vi "HFRR ADV v018 new software.vi"() -> ()   [LabVIEW 2025] (continued)
                }
                frame 126, Default {
                }
              }
            }
          }
          frame #1 {
            w4472 = TRUE ("Visible")
            n3478 = local read "S 91"() -> (w4489:string)
            n3479 = local read "S 90"() -> (w4488:string)
            n3480 = local read "S 88"() -> (w4487:string)
            n3481 = property on="File Path" class="Path"("Caption.Text"=w4488) -> ()  [unwired: 2 in, 2 out]
            n3482 = property on="SrvM CP" class="Bool (strict)"("Boolean Text.Text"=w4487) -> ()  [unwired: 2 in, 2 out]
            n3483 = local read "S 71"() -> (w4482:string)
            n3484 = local read "S 86"() -> (w4484:string)
            n3485 = local read "S 85"() -> (w4485:string)
            n3486 = local read "S 87"() -> (w4483:string)
            n3487 = local read "S 84"() -> (w4486:string)
            n3488 = local read "S 103"() -> (w4471:string)
            n3489 = local read "S 104"() -> (w4470:string)
            n3490 = property on="ENTER THE NEW PASSWORD" class="Str"("Caption.Text"=w4483) -> ()  [unwired: 2 in, 2 out]
            n3491 = property on="Password" class="Str"("Caption.Text"=w4485) -> ()  [unwired: 2 in, 2 out]
            n3492 = property on="ENTER CURRENT PASSWORD" class="Str"("Caption.Text"=w4484) -> ()  [unwired: 2 in, 2 out]
            n3493 = property on="EDIT" class="Bool (strict)"("Boolean Text.Text"=w4482) -> ()  [unwired: 2 in, 2 out]
            n3494 = property on="SAVE" class="Bool (strict)"("Boolean Text.Text"=w4486) -> ()  [unwired: 2 in, 2 out]
            n3495 = Build Array(w4471, w4470) -> (w4469:string[])
            n3496 = property on="Heater Button" class="Bool (strict)"("Strings [4]"=w4469) -> ()  [unwired: 2 in, 2 out]
            n3497 = property on="CH-HUMIDITY WET" class="DigNum (strict)"("Caption.Size to Text?"=w4472) -> ()  [unwired: 2 in, 2 out]
            n3498 = property on="CH-HUMIDITY DRY" class="DigNum (strict)"("Caption.Size to Text?"=w4472) -> ()  [unwired: 2 in, 2 out]
            n3499 = property on="CH-POWER -" class="DigNum (strict)"("Caption.Size to Text?"=w4472) -> ()  [unwired: 2 in, 2 out]
            n3500 = property on="CH-HEATER" class="DigNum (strict)"("Caption.Size to Text?"=w4472) -> ()  [unwired: 2 in, 2 out]
            n3501 = property on="CH-POWER +" class="DigNum (strict)"("Caption.Size to Text?"=w4472) -> ()  [unwired: 2 in, 2 out]
            n3502 = local read "S 92"() -> (w4481:string)
            n3503 = local read "S 93"() -> (w4480:string)
            n3504 = local read "S 105"() -> (w4467:string)
            n3505 = local read "S 106"() -> (w4466:string)
            n3506 = Build Array(w4481, w4480) -> ()  [unwired: 1 out]
            n3507 = Build Array(w4467, w4466) -> (w4468:string[])
            n3508 = local read "S 95"() -> (w4478:string)
            n3509 = local read "S 94"() -> (w4479:string)
            n3510 = local read "bs"() -> (w4494:string)
            n3511 = local read "as"() -> (w4495:string)
            n3512 = property on="Humidity" class="Bool (strict)"("Strings [4]"=w4468) -> ()  [unwired: 2 in, 2 out]
            n3513 = Concatenate Strings(w4494, "\r", w4495) -> ()  [unwired: 1 out]
            n3514 = property on="STROKE GAIN :" class="DigNum (strict)"("Caption.Text"=w4478) -> ()  [unwired: 2 in, 2 out]
            n3515 = property on="DISPLACEMENT :" class="DigNum (strict)"("Caption.Text"=w4479) -> ()  [unwired: 2 in, 2 out]
            n3516 = property on="Rh After" class="DigNum (strict)"("Caption.Size to Text?"=TRUE ("Caption.Size to Text")) -> ()  [unwired: 2 in, 2 out]
            n3517 = local read "S 48"() -> (w4518:string)
            n3518 = local read "S 50"() -> (w4516:string)
            n3519 = local read "S 51"() -> (w4515:string)
            n3520 = local read "S 49"() -> (w4517:string)
            n3521 = local read "S 52"() -> (w4514:string)
            n3522 = local read "as"() -> (w4499:string)
            n3523 = local read "bs"() -> (w4500:string)
            n3524 = local read "S 56"() -> (w4513:string)
            n3525 = local read "S 57"() -> (w4512:string)
            n3526 = local read "S 58"() -> (w4511:string)
            n3527 = local read "S 59"() -> (w4510:string)
            n3528 = property on="OPEN" class="Bool (strict)"("Boolean Text.Text"=w4514) -> ()  [unwired: 2 in, 2 out]
            n3529 = property on="OPEN 1" class="Bool (strict)"("Boolean Text.Text"=w4518) -> ()  [unwired: 2 in, 2 out]
            n3530 = property on="OPEN 2" class="Bool (strict)"("Boolean Text.Text"=w4517) -> ()  [unwired: 2 in, 2 out]
            n3531 = property on="OPEN 3" class="Bool (strict)"("Boolean Text.Text"=w4516) -> ()  [unwired: 2 in, 2 out]
            n3532 = property on="OPEN 4" class="Bool (strict)"("Boolean Text.Text"=w4515) -> ()  [unwired: 2 in, 2 out]
            n3533 = Concatenate Strings(w4500, "\r", w4499) -> ()  [unwired: 1 out]
            n3534 = local read "S 102"() -> (w4473:string)
            n3535 = property on="КОФ1" class="DigNum (strict)"("Caption.Text"=w4513) -> ()  [unwired: 2 in, 2 out]
            n3536 = local read "S 98"() -> (w4477:string)
            n3537 = local read "S 99"() -> (w4476:string)
            n3538 = local read "S 100"() -> (w4475:string)
            n3539 = local read "S 101"() -> (w4474:string)
            n3540 = property on="КОФ2" class="DigNum (strict)"("Caption.Text"=w4512) -> ()  [unwired: 2 in, 2 out]
            n3541 = property on="КОФ3" class="DigNum (strict)"("Caption.Text"=w4511) -> ()  [unwired: 2 in, 2 out]
            n3542 = property on="КОФ4" class="DigNum (strict)"("Caption.Text"=w4510) -> ()  [unwired: 2 in, 2 out]
            n3543 = local read "bs"() -> (w4498:string)
            n3544 = local read "as"() -> (w4497:string)
            n3545 = property on="CH-POWER +" class="DigNum (strict)"("Caption.Text"=w4477) -> ()  [unwired: 2 in, 2 out]
            n3546 = property on="CH-POWER -" class="DigNum (strict)"("Caption.Text"=w4476) -> ()  [unwired: 2 in, 2 out]
            n3547 = property on="CH-HEATER" class="DigNum (strict)"("Caption.Text"=w4475) -> ()  [unwired: 2 in, 2 out]
            n3548 = property on="CH-HUMIDITY DRY" class="DigNum (strict)"("Caption.Text"=w4474) -> ()  [unwired: 2 in, 2 out]
            n3549 = property on="CH-HUMIDITY WET" class="DigNum (strict)"("Caption.Text"=w4473) -> ()  [unwired: 2 in, 2 out]
            n3550 = local read "S 60"() -> (w4509:string)
            n3551 = local read "S 54"() -> (w4519:string)
            n3552 = Concatenate Strings(w4498, "\r", w4497) -> ()  [unwired: 1 out]
            n3553 = Concatenate Strings(w4519, w4509) -> ()  [unwired: 1 out]
            n3554 = local read "S 77"() -> (→"String 43":string)
            n3555 = local read "S 76"() -> (w4492:string)
            n3556 = local read "S 78"() -> (w4491:string)
            n3557 = local read "S 71"() -> (w4503:string)
            n3558 = local read "S 66"() -> (w4508:string)
            n3559 = local read "S 67"() -> (w4507:string)
            n3560 = local read "S 68"() -> (w4506:string)
            n3561 = local read "S 69"() -> (w4505:string)
            n3562 = local read "S 70"() -> (w4504:string)
            n3563 = property on="AIR TEMP" class="DigNum (strict)"("Caption.Text"=w4491) -> ()  [unwired: 2 in, 2 out]
            n3564 = property on="Set Strk" class="DigNum (strict)"("Caption.Text"=w4492) -> ()  [unwired: 2 in, 2 out]
            n3565 = property on="FRIC. FORCE :" class="DigNum (strict)"("Caption.Text"=w4508) -> ()  [unwired: 2 in, 2 out]
            n3566 = property on="TEMPERATURE :" class="DigNum (strict)"("Caption.Text"=w4507) -> ()  [unwired: 2 in, 2 out]
            n3567 = property on="SPEED OUT:" class="DigNum (strict)"("Caption.Text"=w4506) -> ()  [unwired: 2 in, 2 out]
            n3568 = property on="AIR TEMPERATURE :" class="DigNum (strict)"("Caption.Text"=w4505) -> ()  [unwired: 2 in, 2 out]
            n3569 = property on="HUMIDITY:" class="DigNum (strict)"("Caption.Text"=w4504) -> ()  [unwired: 2 in, 2 out]
            n3570 = property on="EDIT" class="Bool (strict)"("Boolean Text.Text"=w4503) -> ()  [unwired: 2 in, 2 out]
            n3571 = local read "S 79"() -> (w4490:string)
          }
          frame #2 {
          }
        }
        n3572 = local write "Lan flag"(10.0 ("Lan flag")) -> ()
      }
      frame Enabled {
      }
    }
    n3573 = Wait (ms)(milliseconds to wait=u32 2000) -> ()  [unwired: 1 out]
    n3574 = local read "Quit"() -> (w4293:bool)
  }
  n3575 = while {
    shift-right: [w4525] -> _
    shift-left: _ -> [w4526]
    shift-right: [w4523] -> _
    shift-left: T18 {"Read Heave and Surge"="", "Bytes at Heave Port"=0.0, "Heave and Surge COM Port:"="COM9", "Com Port 2"="COM7", "Residual Due"="", "Heave COM Status 2"=TRUE, "Heave COM Status"=TRUE, "Port 2"=TRUE, "Sway PPR"=6400.0, "Surge PPR"=6400.0, "Heave PPR"=6400.0, "Sway Pitch"=2.0, "Surge Pitch"=3.0, "Heave Pitch"=4.0, "Sway Pulses/mm"=320.0, "Surge Pulses/mm"=1600.0, "Heave Pulses/mm"=1600.0, "inner loop"=0.0, "Read Heave and Surge 2"="", "String 36"="", "Write S"=FALSE, "WriteCC1"=[""], "Heave COM Loop"=0, "LastCom"="", "EXIT"=FALSE, "Error Heave"={"status"=TRUE, "code"=-1073807343, "source"=""}} -> [w4522]
    shift-right: [w4520] -> _
    shift-left: enum16{"init", "MAIN", "Panel Close"}."init" -> [w4521]
    stop <- w4524 stop-if-true
    n3576 = case shown="\"init\"" w4521 {
      tunnel: w4526 -> [w4540 w4556 w4616 w4618]
      tunnel: [w4535 w4564 w4616 w4618] -> w4525
      tunnel: [_ _ TRUE _] -> w4524
      tunnel: [w4531 w4562 w4614 w4617] -> w4523
      tunnel: w4522 -> [w4537 w4555 w4614 w4617]
      tunnel: [enum16{"init", "MAIN", "Panel Close"}."MAIN" w4550 _ _] -> w4520
      frame "init" {
        n3577 = local read "Com Port 1"() -> (w4527:refnum<visa-resource-name>)
        n3578 = Bundle By Name(cluster=w4537, "Heave and Surge COM Port:"=w4527) -> (w4536:T18)
        n3579 = call "Instrument fgv uno.vi"("Enum"=T31."INIT", "error in (no error) 2"=w4540, "INPUT"=w4536) -> ("error"=w4538:errorcluster, "output"=w4534:T18)  [unwired: 6 in, 1 out]
        n3580 = case shown="Error" w4538 {
          selector: w4538 -> [w4542 _]
          tunnel: [w4542 w4546] -> w4535
          tunnel: w4534 -> [w4541 w4544]
          tunnel: [w4541 w4543] -> w4532
          frame No Error {
          }
          frame Error {
            n3581 = call "Instrument fgv uno.vi"("Enum"=T31."ERROR INIT", "INPUT"=w4544) -> ("error"=w4547:errorcluster, "output"=w4543:T18)  [unwired: 7 in, 1 out]
            n3582 = call <vilib>:"Clear Errors.vi"("error in (no error)"=w4547) -> ("error out"=w4546:errorcluster)  [unwired: 5 in, 1 out]
          }
        }
        n3583 = local read "LastCom 2"() -> (w4530:string)
        n3584 = Unbundle By Name(w4532) -> ("Heave COM Status 2"=→"COM Status 2" →"Instrument Status 2":bool, "Error Heave"=→"Error  2":errorcluster)  [unwired: 1 out]
        n3585 = Bundle By Name(cluster=w4532, "LastCom"=w4530) -> (w4531:T18)
      }
      frame "MAIN" {
        n3586 = Unbundle By Name(w4555) -> ("Com Port 2"=w4566:refnum<visa-resource-name>)
        n3587 = local read "Com Port 1"() -> (w4549:refnum<visa-resource-name>)
        n3588 = local write "Com Port 5"(w4566) -> ()
        n3589 = Bundle By Name(cluster=w4555, "Heave and Surge COM Port:"=w4549) -> (w4554:T18)
        n3590 = Equal?(x=w4566, y=w4549) -> (x = y?=w4565:bool)
        n3591 = case shown="True" w4565 {
          tunnel: [w4570 w4587] -> w4564
          tunnel: w4556 -> [w4571 w4593]
          tunnel: w4554 -> [w4569 w4591]
          tunnel: [w4568 w4586] -> w4562
          frame False {
            n3592 = call <vilib>:"Clear Errors.vi"("error in (no error)"=w4571) -> ("error out"=w4567:errorcluster)  [unwired: 5 in, 1 out]
            n3593 = call "Instrument fgv uno.vi"("Enum"=T31."ERROR INIT", "error in (no error) 2"=w4567, "INPUT"=w4569) -> ("error"=w4573:errorcluster, "output"=w4568:T18)  [unwired: 6 in, 1 out]
            n3594 = call <vilib>:"Clear Errors.vi"("error in (no error)"=w4573) -> ("error out"=w4570:errorcluster)  [unwired: 5 in, 1 out]
          }
          frame True {
            n3595 = call "Instrument fgv uno.vi"("Enum"=T31."READ", "error in (no error) 2"=w4593, "INPUT"=w4591) -> ("error"=w4592:errorcluster, "output"=w4583:T18)  [unwired: 6 in, 1 out]
            n3596 = Bundle By Name(cluster=w4583, "String 36"="String 15") -> (w4582:T18)
            n3597 = case shown="True" "Write S 2" {
              selector: "Write S 2" -> [_ w4613]
              tunnel: w4592 -> [w4606 w4612]
              tunnel: [w4606 w4611] -> w4579
              tunnel: w4582 -> [w4605 w4608]
              tunnel: [w4605 w4607] -> w4578
              frame False {
              }
              frame True {
                n3598 = Not(x=w4613) -> (.not. x?=w4609:bool)
                n3599 = local write "Write S 2"(w4609) -> ()
                n3600 = call "Instrument fgv uno.vi"("Enum"=T31."MANUAL WRITE", "error in (no error) 2"=w4612, "INPUT"=w4608) -> ("error"=w4611:errorcluster, "output"=w4607:T18)  [unwired: 6 in, 1 out]
              }
            }
            n3601 = Array Size(array="WriteHumidity 2") -> (size(s)=w4576:i32)
            n3602 = Greater Than 0?(x=w4576) -> (x > 0?=w4574:bool)
            n3603 = call "Instrument fgv uno.vi"("Enum"=T31."WRITE", "error in (no error) 2"=w4579, "WriteCC1"="WriteHumidity 2", "INPUT"=w4578) -> ("error"=w4589:errorcluster, "WriteCC1 2"=w4577:string[], "output"=w4588:T18)  [unwired: 5 in]
            n3604 = case shown="True" w4574 {
              tunnel: w4577 -> [_ w4595]
              frame False {
              }
              frame True {
                n3605 = local write "WriteHumidity 2"(w4595) -> ()
              }
            }
            n3606 = case shown="No Error" w4589 {
              selector: w4589 -> [w4596 w4599]
              tunnel: w4588 -> [w4597 w4604]
              tunnel: [w4597 w4603] -> w4586
              tunnel: [w4596 w4601] -> w4587
              frame No Error {
              }
              frame Error {
                n3607 = call <vilib>:"Clear Errors.vi"("error in (no error)"=w4599) -> ("error out"=w4598:errorcluster)  [unwired: 5 in, 1 out]
                n3608 = call "Instrument fgv uno.vi"("Enum"=T31."ERROR INIT", "error in (no error) 2"=w4598, "INPUT"=w4604) -> ("error"=w4602:errorcluster, "output"=w4603:T18)  [unwired: 6 in, 1 out]
                n3609 = call <vilib>:"Clear Errors.vi"("error in (no error)"=w4602) -> ("error out"=w4601:errorcluster)  [unwired: 5 in, 1 out]
              }
            }
            n3610 = Unbundle By Name(w4586) -> ("LastCom"=→"LastCom 2":string, "Read Heave and Surge"=→"Read Uno":string)
          }
        }
        n3611 = Unbundle By Name(w4562) -> ("Heave COM Status 2"=w4563:bool, "Heave COM Status"=w4548:bool, "Error Heave"=w4560:errorcluster, "Bytes at Heave Port"=→"Bytes at Humidity Port  2":dbl)
        n3612 = Unbundle By Name(w4560) -> ("status"=→"Humidity Port 2":bool)
        n3613 = Not(x=w4548) -> (.not. x?=w4557:bool)
        n3614 = local write "Error  2"(w4560) -> ()
        n3615 = Not(x=w4563) -> (.not. x?=w4558:bool)
        n3616 = local write "Instrument Status 2"(w4557) -> ()
        n3617 = local write "COM Status 2"(w4558) -> ()
        n3618 = local write "Port 1a"(w4548) -> ()
        n3619 = local read "Quit"() -> (w4551:bool)
        n3620 = Select(t=enum16{"init", "MAIN", "Panel Close"}."Panel Close", s=w4551, f=enum16{"init", "MAIN", "Panel Close"}."MAIN") -> (s? t:f=w4550:enum16{"init", "MAIN", "Panel Close"})
      }
      frame "Panel Close" {
      }
      frame Default {
      }
    }
  }
  n3621 = disable-structure shown="Disabled" {
    frame Disabled {
      n3622 = while {
        tunnel: [w4620] -> _
        i -> [w4620]
        stop <- w4619 continue-if-true
        n3623 = Wait (ms)(milliseconds to wait=u32 50) -> ()  [unwired: 1 out]
        n3624 = stacked-sequence {
          frame #0 {
            # "Controls Text color"
            # "Controls BG color"
            n3625 = property on="FILE" class="Str"("Text.Text Colors:Text Color"="SC  Text") -> ()  [unwired: 2 in, 2 out]
            n3626 = property on="Fuel Discription :" class="Str"("Text.Text Colors:Text Color"="SC  Text") -> ()  [unwired: 2 in, 2 out]
            n3627 = property on="tested by" class="Str"("Text.Text Colors:Text Color"="SC  Text") -> ()  [unwired: 2 in, 2 out]
            n3628 = property on="Remarks :" class="Str"("Text.Text Colors:Text Color"="SC  Text") -> ()  [unwired: 2 in, 2 out]
            n3629 = property class="DigNum (strict)"("Numeric Text.Text Colors:BG Color"="NC BG") -> ()  [unwired: 2 in, 2 out]
            n3630 = property class="DigNum (strict)"("Numeric Text.Text Colors:BG Color"="NC BG") -> ()  [unwired: 2 in, 2 out]
            n3631 = property class="DigNum (strict)"("Numeric Text.Text Colors:BG Color"="NC BG") -> ()  [unwired: 2 in, 2 out]
            n3632 = property class="DigNum (strict)"("Numeric Text.Text Colors:BG Color"="NC BG") -> ()  [unwired: 2 in, 2 out]
            n3633 = property class="DigNum (strict)"("Numeric Text.Text Colors:BG Color"="NC BG") -> ()  [unwired: 2 in, 2 out]
            n3634 = property class="DigNum (strict)"("Numeric Text.Text Colors:BG Color"="NC BG") -> ()  [unwired: 2 in, 2 out]
            n3635 = property class="DigNum (strict)"("Numeric Text.Text Colors:BG Color"="NC BG") -> ()  [unwired: 2 in, 2 out]
            n3636 = property class="DigNum (strict)"("Numeric Text.Text Colors:BG Color"="NC BG") -> ()  [unwired: 2 in, 2 out]
            n3637 = property class="DigNum (strict)"("Numeric Text.Text Colors:BG Color"="NC BG") -> ()  [unwired: 2 in, 2 out]
            n3638 = property class="DigNum (strict)"("Numeric Text.Text Colors:BG Color"="NC BG") -> ()  [unwired: 2 in, 2 out]
            n3639 = property class="DigNum (strict)"("Numeric Text.Text Colors:BG Color"="NC BG") -> ()  [unwired: 2 in, 2 out]
            n3640 = property class="DigNum (strict)"("Numeric Text.Text Colors:BG Color"="NC BG") -> ()  [unwired: 2 in, 2 out]
            n3641 = property on="FILE" class="Str"("Text.Text Colors:BG Color"="SC BG 3") -> ()  [unwired: 2 in, 2 out]
            n3642 = property on="Fuel Discription :" class="Str"("Text.Text Colors:BG Color"="SC BG 3") -> ()  [unwired: 2 in, 2 out]
            n3643 = property on="tested by" class="Str"("Text.Text Colors:BG Color"="SC BG 3") -> ()  [unwired: 2 in, 2 out]
            n3644 = property on="Remarks :" class="Str"("Text.Text Colors:BG Color"="SC BG 3") -> ()  [unwired: 2 in, 2 out]
            n3645 = property class="DigNum (strict)"("Numeric Text.Text Colors:Text Color"="NC Text") -> ()  [unwired: 2 in, 2 out]
            n3646 = property class="DigNum (strict)"("Numeric Text.Text Colors:Text Color"="NC Text") -> ()  [unwired: 2 in, 2 out]
            n3647 = property class="DigNum (strict)"("Numeric Text.Text Colors:Text Color"="NC Text") -> ()  [unwired: 2 in, 2 out]
            n3648 = property class="DigNum (strict)"("Numeric Text.Text Colors:Text Color"="NC Text") -> ()  [unwired: 2 in, 2 out]
            n3649 = property class="DigNum (strict)"("Numeric Text.Text Colors:Text Color"="NC Text") -> ()  [unwired: 2 in, 2 out]
            n3650 = property class="DigNum (strict)"("Numeric Text.Text Colors:Text Color"="NC Text") -> ()  [unwired: 2 in, 2 out]
            n3651 = property class="DigNum (strict)"("Numeric Text.Text Colors:Text Color"="NC Text") -> ()  [unwired: 2 in, 2 out]
            n3652 = property class="DigNum (strict)"("Numeric Text.Text Colors:Text Color"="NC Text") -> ()  [unwired: 2 in, 2 out]
            n3653 = property class="DigNum (strict)"("Numeric Text.Text Colors:Text Color"="NC Text") -> ()  [unwired: 2 in, 2 out]
            n3654 = property class="DigNum (strict)"("Numeric Text.Text Colors:Text Color"="NC Text") -> ()  [unwired: 2 in, 2 out]
            n3655 = property class="DigNum (strict)"("Numeric Text.Text Colors:Text Color"="NC Text") -> ()  [unwired: 2 in, 2 out]
            n3656 = property class="DigNum (strict)"("Numeric Text.Text Colors:Text Color"="NC Text") -> ()  [unwired: 2 in, 2 out]
            n3657 = property class="DigNum (strict)"("Numeric Text.Text Colors:Text Color"="NI Text  2") -> ()  [unwired: 2 in, 2 out]
            n3658 = property class="DigNum (strict)"("Numeric Text.Text Colors:Text Color"="NI Text  2") -> ()  [unwired: 2 in, 2 out]
            n3659 = property class="DigNum (strict)"("Numeric Text.Text Colors:Text Color"="NI Text  2") -> ()  [unwired: 2 in, 2 out]
            n3660 = property class="DigNum (strict)"("Numeric Text.Text Colors:Text Color"="NI Text  2") -> ()  [unwired: 2 in, 2 out]
            n3661 = property class="DigNum (strict)"("Numeric Text.Text Colors:Text Color"="NI Text  2") -> ()  [unwired: 2 in, 2 out]
            n3662 = property class="DigNum (strict)"("Numeric Text.Text Colors:Text Color"="NI Text  2") -> ()  [unwired: 2 in, 2 out]
            n3663 = property class="DigNum (strict)"("Numeric Text.Text Colors:Text Color"="NI Text  2") -> ()  [unwired: 2 in, 2 out]
            n3664 = property class="DigNum (strict)"("Numeric Text.Text Colors:Text Color"="NI Text  2") -> ()  [unwired: 2 in, 2 out]
            n3665 = property class="DigNum (strict)"("Numeric Text.Text Colors:Text Color"="NI Text  2") -> ()  [unwired: 2 in, 2 out]
            n3666 = property class="DigNum (strict)"("Numeric Text.Text Colors:Text Color"="NI Text  2") -> ()  [unwired: 2 in, 2 out]
            n3667 = property class="DigNum (strict)"("Numeric Text.Text Colors:Text Color"="NI Text  2") -> ()  [unwired: 2 in, 2 out]
            n3668 = property class="DigNum (strict)"("Numeric Text.Text Colors:Text Color"="NI Text  2") -> ()  [unwired: 2 in, 2 out]
            n3669 = property class="DigNum (strict)"("Numeric Text.Text Colors:Text Color"="NI Text  2") -> ()  [unwired: 2 in, 2 out]
            n3670 = property class="DigNum (strict)"("Numeric Text.Text Colors:Text Color"="NI Text  2") -> ()  [unwired: 2 in, 2 out]
            n3671 = property class="DigNum (strict)"("Numeric Text.Text Colors:Text Color"="NI Text  2") -> ()  [unwired: 2 in, 2 out]
            n3672 = property on="Coefficient Of Friction" class="XYGraph (strict)"("Plot Area:Colors:FG Color"="GFG  2", "Plot Area:Colors:BG Color"="GBG   2") -> ()  [unwired: 2 in, 2 out]
            n3673 = property on="Humidity ( %RH )" class="XYGraph (strict)"("Plot Area:Colors:FG Color"="GFG  2", "Plot Area:Colors:BG Color"="GBG   2") -> ()  [unwired: 2 in, 2 out]
            n3674 = property on="Air Temperature  ( °C )" class="XYGraph (strict)"("Plot Area:Colors:FG Color"="GFG  2", "Plot Area:Colors:BG Color"="GBG   2") -> ()  [unwired: 2 in, 2 out]
            n3675 = property on="Sample Temperature ( °C )" class="XYGraph (strict)"("Plot Area:Colors:FG Color"="GFG  2", "Plot Area:Colors:BG Color"="GBG   2") -> ()  [unwired: 2 in, 2 out]
            n3676 = property class="DigNum (strict)"("Numeric Text.Text Colors:BG Color"="NI BG 2") -> ()  [unwired: 2 in, 2 out]
            n3677 = property class="DigNum (strict)"("Numeric Text.Text Colors:BG Color"="NI BG 2") -> ()  [unwired: 2 in, 2 out]
            n3678 = property class="DigNum (strict)"("Numeric Text.Text Colors:BG Color"="NI BG 2") -> ()  [unwired: 2 in, 2 out]
            n3679 = property class="DigNum (strict)"("Numeric Text.Text Colors:BG Color"="NI BG 2") -> ()  [unwired: 2 in, 2 out]
            n3680 = property class="DigNum (strict)"("Numeric Text.Text Colors:BG Color"="NI BG 2") -> ()  [unwired: 2 in, 2 out]
            n3681 = property class="DigNum (strict)"("Numeric Text.Text Colors:BG Color"="NI BG 2") -> ()  [unwired: 2 in, 2 out]
            n3682 = property class="DigNum (strict)"("Numeric Text.Text Colors:BG Color"="NI BG 2") -> ()  [unwired: 2 in, 2 out]
            n3683 = property class="DigNum (strict)"("Numeric Text.Text Colors:BG Color"="NI BG 2") -> ()  [unwired: 2 in, 2 out]
            n3684 = property class="DigNum (strict)"("Numeric Text.Text Colors:BG Color"="NI BG 2") -> ()  [unwired: 2 in, 2 out]
            n3685 = property class="DigNum (strict)"("Numeric Text.Text Colors:BG Color"="NI BG 2") -> ()  [unwired: 2 in, 2 out]
            n3686 = property class="DigNum (strict)"("Numeric Text.Text Colors:BG Color"="NI BG 2") -> ()  [unwired: 2 in, 2 out]
            n3687 = property class="DigNum (strict)"("Numeric Text.Text Colors:BG Color"="NI BG 2") -> ()  [unwired: 2 in, 2 out]
            n3688 = property class="DigNum (strict)"("Numeric Text.Text Colors:BG Color"="NI BG 2") -> ()  [unwired: 2 in, 2 out]
            n3689 = property class="DigNum (strict)"("Numeric Text.Text Colors:BG Color"="NI BG 2") -> ()  [unwired: 2 in, 2 out]
            n3690 = property class="DigNum (strict)"("Numeric Text.Text Colors:BG Color"="NI BG 2") -> ()  [unwired: 2 in, 2 out]
            n3691 = property class="Bool"("Colors [4]"="Boolean BC T & BG") -> ()  [unwired: 2 in, 2 out]
            n3692 = property on="Save & Continue" class="Bool (strict)"("Colors [4]"="Boolean BC T & BG") -> ()  [unwired: 2 in, 2 out]
            n3693 = property on="Heater Button" class="Bool (strict)"("Colors [4]"="Boolean BC T & BG") -> ()  [unwired: 2 in, 2 out]
            n3694 = property class="Bool"("Colors [4]"="Boolean BC T & BG") -> ()  [unwired: 2 in, 2 out]
            n3695 = property on="Humidity" class="Bool (strict)"("Colors [4]"="Boolean BC T & BG") -> ()  [unwired: 2 in, 2 out]
            n3696 = property class="Bool (strict)"("Colors [4]"="Boolean BC T & BG") -> ()  [unwired: 2 in, 2 out]
            n3697 = property on="RUN" class="Bool (strict)"("Colors [4]"="Boolean BC T & BG") -> ()  [unwired: 2 in, 2 out]
            n3698 = property on="trip1 8" class="Bool (strict)"("Colors [4]"="Boolean BC T & BG") -> ()  [unwired: 2 in, 2 out]
            n3699 = property class="Bool"("Colors [4]"="Boolean BC T & BG") -> ()  [unwired: 2 in, 2 out]
            n3700 = property class="Bool (strict)"("Colors [4]"="Boolean BC T & BG") -> ()  [unwired: 2 in, 2 out]
            n3701 = property on="OPEN 1" class="Bool (strict)"("Colors [4]"="Boolean BC T & BG 2") -> ()  [unwired: 2 in, 2 out]
            n3702 = property on="OPEN 2" class="Bool (strict)"("Colors [4]"="Boolean BC T & BG 2") -> ()  [unwired: 2 in, 2 out]
            n3703 = property on="OPEN 3" class="Bool (strict)"("Colors [4]"="Boolean BC T & BG 2") -> ()  [unwired: 2 in, 2 out]
            n3704 = property on="OPEN 4" class="Bool (strict)"("Colors [4]"="Boolean BC T & BG 2") -> ()  [unwired: 2 in, 2 out]
            n3705 = property on="OPEN" class="Bool (strict)"("Colors [4]"="Boolean BC T & BG 2") -> ()  [unwired: 2 in, 2 out]
            n3706 = property on="rstv2" class="Bool"("Colors [4]"="Boolean BC T & BG 2") -> ()  [unwired: 2 in, 2 out]
            n3707 = property on="RST CP" class="Bool"("Colors [4]"="Boolean BC T & BG 2") -> ()  [unwired: 2 in, 2 out]
            n3708 = property on="RSTV1 3" class="Bool"("Colors [4]"="Boolean BC T & BG 2") -> ()  [unwired: 2 in, 2 out]
            n3709 = property on="RSTV1 2" class="Bool"("Colors [4]"="Boolean BC T & BG 2") -> ()  [unwired: 2 in, 2 out]
          }
          frame #1 {
          }
        }
        n3710 = local read "Quit"() -> (w4619:bool)
      }
    }
    frame Enabled {
    }
  }
  n3711 = while {
    shift-right: [w4637] -> _
    shift-left: _ -> [w4638]
    shift-right: [w4635] -> _
    shift-left: T18 {"Read Heave and Surge"="", "Bytes at Heave Port"=0.0, "Heave and Surge COM Port:"="COM9", "Com Port 2"="COM7", "Residual Due"="", "Heave COM Status 2"=TRUE, "Heave COM Status"=TRUE, "Port 2"=TRUE, "Sway PPR"=6400.0, "Surge PPR"=6400.0, "Heave PPR"=6400.0, "Sway Pitch"=2.0, "Surge Pitch"=3.0, "Heave Pitch"=4.0, "Sway Pulses/mm"=320.0, "Surge Pulses/mm"=1600.0, "Heave Pulses/mm"=1600.0, "inner loop"=0.0, "Read Heave and Surge 2"="", "String 36"="", "Write S"=FALSE, "WriteCC1"=[""], "Heave COM Loop"=0, "LastCom"="", "EXIT"=FALSE, "Error Heave"={"status"=TRUE, "code"=-1073807343, "source"=""}} -> [w4634]
    shift-right: [w4632] -> _
    shift-left: enum16{"init", "MAIN", "Panel Close"}."init" -> [w4633]
    stop <- w4636 stop-if-true
    n3712 = case shown="\"init\"" w4633 {
      tunnel: w4638 -> [w4652 w4667 w4728 w4730]
      tunnel: [w4646 w4676 w4728 w4730] -> w4637
      tunnel: [_ _ TRUE _] -> w4636
      tunnel: [w4642 w4673 w4726 w4729] -> w4635
      tunnel: w4634 -> [w4649 w4666 w4726 w4729]
      tunnel: [enum16{"init", "MAIN", "Panel Close"}."MAIN" w4660 _ _] -> w4632
      frame "init" {
        n3713 = Bundle By Name(cluster=w4649, "Heave and Surge COM Port:"="C3 :") -> (w4648:T18)
        n3714 = call "Instrument fgv.vi"("Enum"=T31."INIT", "error in (no error) 2"=w4652, "INPUT"=w4648) -> ("error"=w4650:errorcluster, "output"=w4645:T18)  [unwired: 6 in, 1 out]
        n3715 = case shown="Error" w4650 {
          selector: w4650 -> [w4654 _]
          tunnel: [w4654 w4658] -> w4646
          tunnel: w4645 -> [w4653 w4656]
          tunnel: [w4653 w4655] -> w4643
          frame No Error {
          }
          frame Error {
            n3716 = call "Instrument fgv.vi"("Enum"=T31."ERROR INIT", "INPUT"=w4656) -> ("error"=w4659:errorcluster, "output"=w4655:T18)  [unwired: 7 in, 1 out]
            n3717 = call <vilib>:"Clear Errors.vi"("error in (no error)"=w4659) -> ("error out"=w4658:errorcluster)  [unwired: 5 in, 1 out]
          }
        }
        n3718 = local read "LastCom"() -> (w4641:string)
        n3719 = Unbundle By Name(w4643) -> ("Heave COM Status 2"=→"COM Status" →"Instrument Status":bool, "Error Heave"=→"Error":errorcluster)  [unwired: 1 out]
        n3720 = Bundle By Name(cluster=w4643, "LastCom"=w4641) -> (w4642:T18)
      }
      frame "MAIN" {
        n3721 = Unbundle By Name(w4666) -> ("Com Port 2"=w4678:refnum<visa-resource-name>)
        n3722 = local write "Com Port 4"(w4678) -> ()
        n3723 = local read "C3 :"() -> (w4664:refnum<visa-resource-name>)
        n3724 = Bundle By Name(cluster=w4666, "Heave and Surge COM Port:"=w4664) -> (w4665:T18)
        n3725 = Equal?(x=w4678, y=w4664) -> (x = y?=w4677:bool)
        n3726 = case shown="True" w4677 {
          tunnel: [w4682 w4699] -> w4676
          tunnel: w4667 -> [w4683 w4705]
          tunnel: w4665 -> [w4681 w4703]
          tunnel: [w4680 w4698] -> w4673
          frame False {
            n3727 = call <vilib>:"Clear Errors.vi"("error in (no error)"=w4683) -> ("error out"=w4679:errorcluster)  [unwired: 5 in, 1 out]
            n3728 = call "Instrument fgv.vi"("Enum"=T31."ERROR INIT", "error in (no error) 2"=w4679, "INPUT"=w4681) -> ("error"=w4685:errorcluster, "output"=w4680:T18)  [unwired: 6 in, 1 out]
            n3729 = call <vilib>:"Clear Errors.vi"("error in (no error)"=w4685) -> ("error out"=w4682:errorcluster)  [unwired: 5 in, 1 out]
          }
          frame True {
            n3730 = call "Instrument fgv.vi"("Enum"=T31."READ", "error in (no error) 2"=w4705, "INPUT"=w4703) -> ("error"=w4704:errorcluster, "output"=w4695:T18)  [unwired: 6 in, 1 out]
            n3731 = Bundle By Name(cluster=w4695, "String 36"="String 11") -> (w4694:T18)
            n3732 = case shown="True" "Write S" {
              selector: "Write S" -> [_ w4725]
              tunnel: w4704 -> [w4718 w4724]
              tunnel: [w4718 w4723] -> w4691
              tunnel: w4694 -> [w4717 w4720]
              tunnel: [w4717 w4719] -> w4690
              frame False {
              }
              frame True {
                n3733 = Not(x=w4725) -> (.not. x?=w4721:bool)
                n3734 = local write "Write S"(w4721) -> ()
                n3735 = call "Instrument fgv.vi"("Enum"=T31."MANUAL WRITE", "error in (no error) 2"=w4724, "INPUT"=w4720) -> ("error"=w4723:errorcluster, "output"=w4719:T18)  [unwired: 6 in, 1 out]
              }
            }
            n3736 = Array Size(array="WriteHumidity") -> (size(s)=w4688:i32)
            n3737 = Greater Than 0?(x=w4688) -> (x > 0?=w4686:bool)
            n3738 = call "Instrument fgv.vi"("Enum"=T31."WRITE", "error in (no error) 2"=w4691, "WriteCC1"="WriteHumidity", "INPUT"=w4690) -> ("error"=w4701:errorcluster, "WriteCC1 2"=w4689:string[], "output"=w4700:T18)  [unwired: 5 in]
            n3739 = case shown="True" w4686 {
              tunnel: w4689 -> [_ w4707]
              frame False {
              }
              frame True {
                n3740 = local write "WriteHumidity"(w4707) -> ()
              }
            }
            n3741 = case shown="Error" w4701 {
              selector: w4701 -> [w4708 w4711]
              tunnel: w4700 -> [w4709 w4716]
              tunnel: [w4709 w4715] -> w4698
              tunnel: [w4708 w4713] -> w4699
              frame No Error {
              }
              frame Error {
                n3742 = call <vilib>:"Clear Errors.vi"("error in (no error)"=w4711) -> ("error out"=w4710:errorcluster)  [unwired: 5 in, 1 out]
                n3743 = call "Instrument fgv.vi"("Enum"=T31."ERROR INIT", "error in (no error) 2"=w4710, "INPUT"=w4716) -> ("error"=w4714:errorcluster, "output"=w4715:T18)  [unwired: 6 in, 1 out]
                n3744 = call <vilib>:"Clear Errors.vi"("error in (no error)"=w4714) -> ("error out"=w4713:errorcluster)  [unwired: 5 in, 1 out]
              }
            }
            n3745 = Unbundle By Name(w4698) -> ("LastCom"=→"LastCom":string, "Read Heave and Surge"=→"Read Humidity":string)
          }
        }
        n3746 = Unbundle By Name(w4673) -> ("Heave COM Status 2"=w4675:bool, "Heave COM Status"=w4674:bool, "Error Heave"=w4671:errorcluster, "Bytes at Heave Port"=→"Bytes at Humidity Port":dbl)
        n3747 = Unbundle By Name(w4671) -> ("status"=→"Humidity Port":bool)
        n3748 = Not(x=w4674) -> (.not. x?=w4668:bool)
        n3749 = local write "Error"(w4671) -> ()
        n3750 = Not(x=w4675) -> (.not. x?=w4669:bool)
        n3751 = local write "Instrument Status"(w4668) -> ()
        n3752 = local write "COM Status"(w4669) -> ()
        n3753 = local read "Quit"() -> (w4661:bool)
        n3754 = Select(t=enum16{"init", "MAIN", "Panel Close"}."Panel Close", s=w4661, f=enum16{"init", "MAIN", "Panel Close"}."MAIN") -> (s? t:f=w4660:enum16{"init", "MAIN", "Panel Close"})
      }
      frame "Panel Close" {
      }
      frame Default {
      }
    }
  }
  n3755 = while {
    stop <- w4756 stop-if-true
    n3756 = local read "Read Humidity"() -> (w4737:string)
    n3757 = call <vilib>:"High Resolution Polling Wait.vi"("seconds to wait"=0.05) -> ()  [unwired: 10 in, 1 out]
    n3758 = Spreadsheet String To Array(delimiter (Tab)=",", format string="", spreadsheet string=w4737, array type (2D Dbl)=string[] []) -> (array=w4751:string[])
    n3759 = for {
      tunnel: w4751 -> [w4761] mode=indexing
      tunnel: string[] ["STATE;", "SET;", "RH;", "T;", "AMB_RH;", "AMB_T;", "PUMP;", "FAN_IN;", "FAN_OUT;", "DEHUM;", "CURRENT;", "STALL;"] -> [w4760] mode=indexing
      tunnel: [w4759] -> w4750 mode=indexing
      n3760 = Match Pattern(string=w4761, regular expression=w4760) -> (after substring=w4759:string)  [unwired: 1 in, 3 out]
    }
    n3761 = Index Array(array=w4750) -> (element #1=→"STATE :":string, element #2=→"SET :":string, element #3=w4739:string, element #4=→"T :":string, element #5=w4736:string, element #6=→"AMB_T :":string, element #7=→"PUMP :":string, element #8=→"FAN_IN :":string, element #9=→"FAN_OUT :":string, element #10=→"DEHUM :":string, element #11=→"CURRENT :":string, element #12=→"STALL :":string)  [unwired: 12 in]
    "RH :" <- w4739
    "AMB_RH :" <- w4736
    n3762 = Fract/Exp String To Number(string=w4739) -> (number=w4731:dbl)  [unwired: 3 in, 1 out]
    n3763 = Fract/Exp String To Number(string=w4736) -> (number=w4735:dbl)  [unwired: 3 in, 1 out]
    n3764 = local write "Ambient Humidity :"(w4735) -> ()
    n3765 = Equal?(x=w4731, y=0.0) -> (x = y?=w4733:bool)
    n3766 = case shown="True" w4733 {
      tunnel: [w4757 w4758] -> w4732
      tunnel: w4731 -> [w4757 _]
      frame False {
        (unwired) 0.0
        "Humidity temp" <- w4757
      }
      frame True {
        n3767 = local read "Humidity temp"() -> (w4758:dbl)
      }
    }
    "RH Numeric:" <- w4732
    n3768 = local read "Quit"() -> (w4756:bool)
  }
  n3769 = disable-structure shown="Disabled" {
    frame Disabled {
      n3770 = while {
        tunnel: [w4995] -> _
        i -> [w4995]
        stop <- w4992 stop-if-true
        n3771 = local read "powstat"() -> (w4993:bool)
        n3772 = case shown="True" w4993 {
          frame False {
          }
          frame True {
            n3773 = local read "RUN"() -> (w4996:bool)
            n3774 = case shown="True" w4996 {
              frame False {
                w5026 = 65.0 ("y")
                n3775 = local read "Set Hz"() -> (w5054:dbl)
                n3776 = local read "NORMAL LOAD"() -> (w5055:dbl)
                n3777 = Multiply(x=w5054, y=60.0) -> (x*y=w5061:dbl)
                n3778 = Multiply(x=1.2 ("y"), y=0.949) -> (x*y=w5030:dbl)
                n3779 = Multiply(x=1.2 ("y"), y=0.8166) -> (x*y=w5034:dbl)
                n3780 = Multiply(x=1.2 ("y"), y=0.851) -> (x*y=w5029:dbl)
                n3781 = local read "FF 2"() -> (w5053:dbl)
                n3782 = Absolute Value(x=w5061) -> (abs(x)=w5059:dbl)
                n3783 = case shown="13.." w5053 {
                  tunnel: [1 2 3] -> w5051
                  frame 0..10, Default {
                    # "Normal"
                  }
                  frame 11, 12 {
                  }
                  frame 13.. {
                  }
                }
                "FF STATE" <- w5051
                n3784 = local read "TEMP"() -> (w5014:dbl)
                n3785 = local read item#-1() -> (w5028)
                n3786 = Less?(x=w5028, y=w5034) -> (x < y?=w5031:bool)
                n3787 = In Range and Coerce(upper limit=w5030, x=w5028, lower limit=w5029) -> (In Range?=w5032:bool)  [unwired: 1 out]
                n3788 = case shown="3601.." w5059 {
                  tunnel: [1 2 3] -> w5057
                  frame 0..3000, Default {
                    # "Normal"
                  }
                  frame 3001..3600 {
                  }
                  frame 3601.. {
                  }
                }
                n3789 = case shown="11.." w5055 {
                  tunnel: [1 3] -> w5056
                  frame 1..10, Default {
                  }
                  frame 11.. {
                  }
                }
                "NL STATE" <- w5056
                n3790 = Multiply(x=1.2 ("y"), y=0.95) -> (x*y=w5044:dbl)
                n3791 = Multiply(x=w5026, y=0.954) -> (x*y=w5018:dbl)
                n3792 = Or(x=w5031, y=w5032) -> (x .or. y?=w5033:bool)
                n3793 = Greater Or Equal?(x=w5028, y=w5044) -> (x >= y?=w5041:bool)
                n3794 = Multiply(x=w5026, y=0.99) -> (x*y=w5015:dbl)
                n3795 = Greater Or Equal?(x=w5014, y=w5015) -> (x >= y?=w5020:bool)
                n3796 = Greater Or Equal?(x=w5014, y=w5018) -> (x >= y?=w5017:bool)
                n3797 = case shown="0, 1, Default" w5028 {
                  tunnel: [1 3] -> w5045
                  frame 0, 1, Default {
                  }
                  frame 2.. {
                  }
                }
                n3798 = case shown="True" w5041 {
                  tunnel: [1 3] -> w5046
                  frame False {
                  }
                  frame True {
                  }
                }
                n3799 = case shown="True" w5033 {
                  tunnel: [1 2] -> w5047
                  frame False {
                  }
                  frame True {
                  }
                }
                n3800 = case shown="..0" w5014 {
                  tunnel: [2 3 3 1] -> w5021
                  frame 61, 62 {
                  }
                  frame 63.. {
                  }
                  frame ..0 {
                  }
                  frame 10..60, Default {
                  }
                }
                n3801 = case shown="True" w5020 {
                  tunnel: [1 3] -> w5022
                  frame False {
                  }
                  frame True {
                  }
                }
                n3802 = Number To Decimal String(number=w5057) -> (decimal integer string=w5058:string)  [unwired: 1 in]
                n3803 = case shown="True" w5017 {
                  tunnel: [1 2] -> w5023
                  frame False {
                  }
                  frame True {
                  }
                }
                n3804 = Number To Decimal String(number=1) -> (decimal integer string=→"Air temp":string)  [unwired: 1 in]
                n3805 = Number To Decimal String(number=w5051) -> (decimal integer string=→"ff_st":string)  [unwired: 1 in]
                n3806 = local write "sp_st"(w5058) -> ()
                n3807 = Number To Decimal String(number=w5056) -> (decimal integer string=→"nl_st":string)  [unwired: 1 in]
                n3808 = Build Array(w5021, w5022, w5023) -> (w5024:i32[])
                n3809 = Build Array(w5045, w5046, w5047) -> (w5048:i32[])
                n3810 = Array Max & Min(array=w5024) -> (max value=w5025:i32)  [unwired: 3 out]
                n3811 = Array Max & Min(array=w5048) -> (max value=w5049:i32)  [unwired: 3 out]
                n3812 = Number To Decimal String(number=w5025) -> (decimal integer string=w5013:string)  [unwired: 1 in]
                n3813 = Number To Decimal String(number=w5049) -> (decimal integer string=→"Stroke Ln 2":string)  [unwired: 1 in]
                n3814 = local write "temp_st"(w5013) -> ()
              }
              frame True {
                w5111 = 65.0 ("y")
                # "Healthy -1\nWarning -2\nError -3"
                n3815 = local read "TEMP"() -> (w5122:dbl)
                n3816 = local read "NORMAL LOAD"() -> (w5126:dbl)
                n3817 = local read "Set Hz"() -> (w5124:dbl)
                n3818 = Multiply(x=1.2 ("y"), y=0.949) -> (x*y=w5106:dbl)
                n3819 = Multiply(x=1.2 ("y"), y=0.8166) -> (x*y=w5102:dbl)
                n3820 = Multiply(x=1.2 ("y"), y=0.851) -> (x*y=w5107:dbl)
                n3821 = Multiply(x=w5111, y=0.954) -> (x*y=w5118:dbl)
                n3822 = Multiply(x=w5111, y=0.99) -> (x*y=w5121:dbl)
                n3823 = Greater Or Equal?(x=w5122, y=w5121) -> (x >= y?=w5116:bool)
                n3824 = Multiply(x=w5124, y=60.0) -> (x*y=w5130:dbl)
                n3825 = Greater Or Equal?(x=w5122, y=w5118) -> (x >= y?=w5119:bool)
                n3826 = local read "FF 2"() -> (w5125:dbl)
                n3827 = local read item#-1() -> (w5108)
                n3828 = Less?(x=w5108, y=w5102) -> (x < y?=w5105:bool)
                n3829 = In Range and Coerce(upper limit=w5106, x=w5108, lower limit=w5107) -> (In Range?=w5104:bool)  [unwired: 1 out]
                n3830 = Absolute Value(x=w5130) -> (abs(x)=w5128:dbl)
                n3831 = case shown="63.." w5122 {
                  tunnel: [2 3 3 1] -> w5115
                  frame 61, 62 {
                  }
                  frame 63.. {
                  }
                  frame ..0 {
                  }
                  frame 10..60, Default {
                  }
                }
                n3832 = case shown="True" w5116 {
                  tunnel: [1 3] -> w5114
                  frame False {
                  }
                  frame True {
                  }
                }
                n3833 = case shown="True" w5119 {
                  tunnel: [1 2] -> w5113
                  frame False {
                  }
                  frame True {
                  }
                }
                n3834 = Multiply(x=1.2 ("y"), y=0.95) -> (x*y=w5092:dbl)
                n3835 = case shown="1..10, Default" w5126 {
                  tunnel: [1 3] -> w5133
                  frame 1..10, Default {
                  }
                  frame 11.. {
                  }
                }
                n3836 = case shown="0..10, Default" w5125 {
                  tunnel: [1 2 3] -> w5132
                  frame 0..10, Default {
                  }
                  frame 11, 12 {
                  }
                  frame 13.. {
                  }
                }
                n3837 = case shown="3601.." w5128 {
                  tunnel: [1 2 3] -> w5127
                  frame 0..3000, Default {
                    # "Normal"
                  }
                  frame 3001..3600 {
                  }
                  frame 3601.. {
                  }
                }
                n3838 = Or(x=w5105, y=w5104) -> (x .or. y?=w5103:bool)
                n3839 = Greater Or Equal?(x=w5108, y=w5092) -> (x >= y?=w5095:bool)
                n3840 = case shown="0, 1, Default" w5108 {
                  tunnel: [1 3] -> w5091
                  frame 0, 1, Default {
                  }
                  frame 2.. {
                  }
                }
                n3841 = case shown="True" w5095 {
                  tunnel: [1 3] -> w5090
                  frame False {
                  }
                  frame True {
                  }
                }
                n3842 = case shown="True" w5103 {
                  tunnel: [1 2] -> w5089
                  frame False {
                  }
                  frame True {
                  }
                }
                n3843 = Build Array(w5115, w5114, w5113) -> (w5112:i32[])
                n3844 = Number To Decimal String(number=w5127) -> (decimal integer string=→"sp_st":string)  [unwired: 1 in]
                n3845 = Array Max & Min(array=w5112) -> (max value=w5109:i32)  [unwired: 3 out]
                "TEMP STATE" <- w5109
                n3846 = Number To Decimal String(number=w5133) -> (decimal integer string=w5136:string)  [unwired: 1 in]
                n3847 = Number To Decimal String(number=w5132) -> (decimal integer string=w5134:string)  [unwired: 1 in]
                n3848 = Number To Decimal String(number=w5109) -> (decimal integer string=→"temp_st":string)  [unwired: 1 in]
                n3849 = Build Array(w5091, w5090, w5089) -> (w5088:i32[])
                n3850 = local write "nl_st"(w5136) -> ()
                n3851 = local write "ff_st"(w5134) -> ()
                n3852 = Number To Decimal String(number=1) -> (decimal integer string=w5131:string)  [unwired: 1 in]
                n3853 = Array Max & Min(array=w5088) -> (max value=w5087:i32)  [unwired: 3 out]
                n3854 = local write "Air temp"(w5131) -> ()
                n3855 = Number To Decimal String(number=w5087) -> (decimal integer string=w5086:string)  [unwired: 1 in]
                n3856 = local write "Stroke Ln 2"(w5086) -> ()
              }
            }
            n3857 = local read "Stroke Ln 2"() -> (w4998:string)
            n3858 = local read "nl_st"() -> (w5004:string)
            n3859 = local read "ff_st"() -> (w5001:string)
            n3860 = local read "sp_st"() -> (w5002:string)
            n3861 = local read "temp_st"() -> (w5003:string)
            n3862 = local read "Air temp"() -> (w4997:string)
            n3863 = Replace Array Subset(array="in", new element #1=w5004, index #1=1 ("index"), new element #2=w5001, index #2=2 ("index"), new element #3=w5003, index #3=3 ("index"), new element #4=w5002, index #4=4 ("index"), new element #5=w4998, index #5=5 ("index"), new element #6=w4997, index #6=6 ("index"), new element #7="Sensor State" ("new element/subarray"), index #7=0 ("index")) -> (→"out":string[])
          }
        }
        n3864 = Wait (ms)(milliseconds to wait=u32 10) -> ()  [unwired: 1 out]
        n3865 = local read "Quit"() -> (w4992:bool)
      }
      n3866 = while {
        stop <- w4967 stop-if-true
        n3867 = local read "run replace"() -> (w4969:bool)
        n3868 = Wait (ms)(milliseconds to wait=u32 100) -> ()  [unwired: 1 out]
        n3869 = Equal?(x="FLAG 2", y=0.0) -> (x = y?=w4970:bool)
        n3870 = case shown="True" w4970 {
          frame False {
          }
          frame True {
            n3871 = local write "FLAG 2"(100.0 ("FLAG 2")) -> ()
            n3872 = call <vilib>:"Read Characters From File.vi"("file path (dialog if empty)"=path "C:/LAB-IQ-NXT/WO 2449 TT.sig", "convert eol? (no:F)"=FALSE ("append to file? (new file:F)")) -> ("character string"=w4973:string)  [unwired: 4 in, 3 out]
            n3873 = call <vilib>:"Read Characters From File.vi"("file path (dialog if empty)"=path "C:/LAB-IQ-NXT/WO 2449 TRH.sig", "convert eol? (no:F)"=FALSE ("append to file? (new file:F)")) -> ("character string"=w4974:string)  [unwired: 4 in, 3 out]
            n3874 = Decimal String To Number(string=w4973) -> (number=w4975:i32)  [unwired: 2 in, 1 out]
            n3875 = local write "Total No. of Tests"(w4975) -> ()
            n3876 = Decimal String To Number(string=w4974) -> (number=w4978:i32)  [unwired: 2 in, 1 out]
            n3877 = local write "SEN.RUN HRS"(w4978) -> ()
          }
        }
        n3878 = case shown="True" w4969 {
          frame False {
          }
          frame True {
            n3879 = Equal?(x="FLAG 4", y=0.0) -> (x = y?=w4982:bool)
            n3880 = case shown="False" w4982 {
              frame False {
                n3881 = Get Date/Time In Seconds() -> (seconds since 1Jan1904=w4988:timestamp)
                n3882 = local read "START 3"() -> (w4986:dbl)
                n3883 = To Double Precision Float(number=w4988) -> (double precision float=w4987:dbl)
                n3884 = Subtract(x=w4987, y=w4986) -> (x-y=→"SENSOR TIME":dbl)
              }
              frame True {
                n3885 = Get Date/Time In Seconds() -> (seconds since 1Jan1904=w4990:timestamp)
                n3886 = local write "FLAG 4"(100.0 ("FLAG")) -> ()
                n3887 = To Double Precision Float(number=w4990) -> (double precision float=→"START 3":dbl)
              }
            }
          }
        }
        n3888 = local read "Quit"() -> (w4967:bool)
      }
      n3889 = while {
        shift-right: [w4767] -> _
        shift-left: _ -> [w4768]
        tunnel: [w4763] -> _
        i -> [w4763]
        stop <- w4762 stop-if-true
        n3890 = Wait (ms)(milliseconds to wait=u32 50 ("Refresh Rate (ms)")) -> ()  [unwired: 1 out]
        n3891 = local read "Json End Flg"() -> (w4764:bool)
        n3892 = Not(x="Upld AR 2") -> ()  [unwired: 1 out]
        n3893 = local read "Upld AR 2"() -> (w4765:bool)
        n3894 = call "Elapsed Time9"("Time Target (s)"="Sen.Upload Rate (s)", "Reset"=FALSE, "Auto Reset"=TRUE) -> ("Time has Elapsed"=w4774:bool)  [unwired: 9 in, 7 out]
        n3895 = Or(x=w4774, y=w4764) -> (x .or. y?=w4770:bool)
        n3896 = case shown="True" w4770 {
          frame False {
          }
          frame True {
            w4866 = "\"SensorName\":\"" ("string")
            w4836 = " \"},{"
            w4861 = "\",\"SensorState\":\""
            w4863 = "\",\"SensorModelNumber\":\"" ("string")
            w4862 = "\",\"SensorRuntimeHours\":\"" ("string")
            n3897 = local read "model num"() -> (w4860:string[])
            n3898 = local read "Sensor name"() -> (w4879:string[])
            n3899 = local read "run"() -> (w4850:string[])
            n3900 = local read "SENSOR TIME"() -> (w4806:dbl)
            n3901 = local read "out"() -> (w4799:string[])
            n3902 = local read "Total No. of Tests"() -> (w4804:dbl)
            n3903 = Select(t=60.0, s="Run test 3", f=3600.0) -> (s? t:f=w4814:dbl)
            n3904 = Index Array(array=w4860, index #1=1 ("index")) -> (element #1=w4859:string, element #2=w4858:string, element #3=w4857:string, element #4=w4856:string, element #5=w4855:string, element #6=w4854:string)  [unwired: 5 in]
            n3905 = Index Array(array=w4850, index #1=1 ("index")) -> (element #1=w4849:string, element #2=w4848:string, element #3=w4847:string, element #4=w4846:string, element #5=w4845:string, element #6=w4844:string)  [unwired: 5 in]
            n3906 = Index Array(array=w4879, index #1=1 ("index")) -> (element #1=w4878:string, element #2=w4877:string, element #3=w4876:string, element #4=w4875:string, element #5=w4865:string, element #6=w4864:string)  [unwired: 5 in]
            n3907 = Index Array(array=w4799, index #1=1 ("index")) -> (element #1=w4831:string, element #2=w4830:string, element #3=w4829:string, element #4=w4828:string, element #5=w4827:string, element #6=w4826:string)  [unwired: 5 in]
            n3908 = local read "SEN.RUN HRS"() -> (w4802:dbl)
            n3909 = Divide(x=w4806, y=w4814) -> (x/y=w4813:dbl)
            n3910 = Increment(x=w4813) -> (x+1=w4809:dbl)
            n3911 = Number To Decimal String(number=w4809) -> (decimal integer string=→"run hrs":string)  [unwired: 1 in]
            n3912 = Divide(x=w4802, y=3600.0 ("f")) -> (x/y=w4797:dbl)
            n3913 = Round To Nearest(number=w4797) -> (nearest integer value=w4795:dbl)
            n3914 = Number To Decimal String(number=w4795) -> (decimal integer string=w4796:string)  [unwired: 1 in]
            n3915 = Number To Decimal String(number=w4804) -> (decimal integer string=w4805:string)  [unwired: 1 in]
            n3916 = local read "Model No"() -> (w4810:string)
            n3917 = local read "UUID"() -> (w4905:string)
            n3918 = local read "Serial No"() -> (w4909:string)
            n3919 = local read "Secret Key"() -> (w4910:string)
            n3920 = Concatenate Strings("\",\"MachineSerialNumber\":\"" ("string"), w4909) -> (w4913:string)
            n3921 = Concatenate Strings("\",\"ModelNumber\":\"" ("string"), w4810) -> (w4811:string)
            n3922 = Concatenate Strings("\",\"MachineRuntimeHours\":\"" ("string"), w4796) -> (w4914:string)
            n3923 = Concatenate Strings("\",\"MachineRuntimeCycles\":\"", w4805) -> (w4907:string)
            n3924 = Concatenate Strings(w4863, w4859) -> (w4893:string)
            n3925 = Concatenate Strings(w4862, w4849) -> (w4894:string)
            n3926 = Concatenate Strings(w4861, w4831) -> (w4892:string)
            n3927 = Concatenate Strings(w4913, w4811, w4914, w4907) -> (w4916:string)
            n3928 = Concatenate Strings(w4863, w4858) -> (w4890:string)
            n3929 = Concatenate Strings(w4862, w4848) -> (w4889:string)
            n3930 = Concatenate Strings(w4861, w4830) -> (w4891:string)
            n3931 = Concatenate Strings(w4863, w4857) -> (w4885:string)
            n3932 = Concatenate Strings(w4862, w4847) -> (w4886:string)
            n3933 = Concatenate Strings(w4861, w4829) -> (w4884:string)
            n3934 = Concatenate Strings(w4863, w4856) -> (w4882:string)
            n3935 = Concatenate Strings(w4862, w4846) -> (w4881:string)
            n3936 = Concatenate Strings(w4861, w4828) -> (w4883:string)
            n3937 = Concatenate Strings(w4893, w4894, w4892) -> (w4895:string)
            n3938 = Concatenate Strings(w4863, w4855) -> (w4872:string)
            n3939 = Concatenate Strings(w4862, w4845) -> (w4873:string)
            n3940 = Concatenate Strings(w4863, w4854) -> (w4869:string)
            n3941 = Concatenate Strings(w4862, w4844) -> (w4868:string)
            n3942 = Concatenate Strings(w4861, w4827) -> (w4871:string)
            n3943 = Concatenate Strings(w4861, w4826) -> (w4870:string)
            n3944 = Concatenate Strings("{\"SecretKey\":\"", w4910, w4916, "\",\"UUID\" : \"", w4905, "\",\"SensorInformation\":", "[{" ("string")) -> (w4843:string)
            n3945 = Concatenate Strings(w4890, w4889, w4891) -> (w4888:string)
            n3946 = Concatenate Strings(w4885, w4886, w4884) -> (w4887:string)
            n3947 = Concatenate Strings(w4882, w4881, w4883) -> (w4880:string)
            n3948 = Concatenate Strings(w4872, w4873, w4871) -> (w4874:string)
            n3949 = Concatenate Strings(w4869, w4868, w4870) -> (w4867:string)
            n3950 = Concatenate Strings(w4866, w4878, w4895, w4836) -> (w4842:string)
            n3951 = Concatenate Strings(w4866, w4877, w4888, w4836) -> (w4841:string)
            n3952 = Concatenate Strings(w4866, w4876, w4887, w4836) -> (w4840:string)
            n3953 = Concatenate Strings(w4866, w4875, w4880, w4836) -> (w4839:string)
            n3954 = Concatenate Strings(w4866, w4865, w4874, w4836) -> (w4838:string)
            n3955 = Concatenate Strings(w4866, w4864, w4867, "\"}" ("string")) -> (w4837:string)
            n3956 = Concatenate Strings(w4843, w4842, w4841, w4840, w4839, w4838, w4837, "]}" ("string")) -> (w4834:string)
            n3957 = local read "SEN.RUN HRS"() -> (w4801:dbl)
            n3958 = disable-structure shown="Disabled" {
              frame Disabled {
                n3959 = local read "state"() -> (w4920:string[])
                n3960 = Delete From Array(array=w4920, index=0) -> (array with subset deleted=w4918:string[])  [unwired: 1 in, 1 out]
                n3961 = for {
                  N: 6 -> [_]
                  tunnel: w4918 -> [w4931] mode=indexing
                  tunnel: [w4930] -> w4917 mode=indexing
                  n3962 = Equal?(x=w4931, y="Warning") -> (x = y?=w4927:bool)
                  n3963 = Equal?(x=w4931, y="Healthy") -> (x = y?=w4924:bool)
                  n3964 = Select(t="2" ("y"), s=w4927, f="3" ("y")) -> (s? t:f=w4922:string)
                  n3965 = Select(t="1" ("y"), s=w4924, f=w4922) -> (s? t:f=w4930:string)
                }
                "state1" <- w4917
              }
              frame Enabled {
              }
            }
            n3966 = stacked-sequence {
              tunnel: w4834 -> [w4942 _ _]
              tunnel: [_ _ w4958] -> _
              frame #0 {
                (unwired) FALSE ("convert eol (F)")
                w4944 = enum16{"start", "end", "current"}."start" ("pos mode (0:2)")
                n3967 = local read "Path"() -> (w4938:path)
                n3968 = Path To String(path=w4938) -> (string=w4950:string)
                n3969 = Concatenate Strings(w4950, "\\", "Sensor File Name") -> (w4951:string)
                n3970 = local write "standard output 2"(" ") -> ()
                n3971 = String To Path(string=w4951) -> (path=w4941:path)
                n3972 = call <vilib>:"Open_Create_Replace File.vi"("advisory dialog? (display:T)"=FALSE, "function (open:0)"=T32."create or replace", "file path"=w4941) -> ("error out"=w4954:errorcluster, "refnum"=w4953:refnum<file>)  [unwired: 5 in, 2 out]
                n3973 = Set File Position(refnum=w4953, from (0:start)=w4944, error in=w4954) -> (refnum out=w4934:refnum<file>, error out=w4933:errorcluster)  [unwired: 1 in]
                n3974 = Write to Binary File(file (use dialog)=w4934, data=" ", error in=w4933, 5:FALSE ("prepend array or string size? (T)")) -> (refnum out=w4945:refnum<file>, error out=w4946:errorcluster)  [unwired: 2 in, 1 out]
                n3975 = Set File Position(offset (in bytes) (0)=w4944, refnum=w4945, error in=w4946) -> (refnum out=w4937:refnum<file>, error out=w4936:errorcluster)  [unwired: 1 in]
                n3976 = Write to Binary File(file (use dialog)=w4937, data=w4942, error in=w4936, 5:FALSE ("prepend array or string size? (T)")) -> (error out=w4940:errorcluster)  [unwired: 2 in, 2 out]
                n3977 = flat-sequence {
                  tunnel: w4941 -> [w4956]
                  tunnel: w4940 -> [_]
                  frame #0 {
                    n3978 = call <vilib>:"Read Characters From File.vi"("file path (dialog if empty)"=w4956) -> ("character string"=→"Sensor Health JSON string":string)  [unwired: 5 in, 3 out]
                  }
                }
                "SinglePoint  2" <- w4942
              }
              frame #1 {
              }
              frame #2 {
                (unwired) "\"Stored\": true" ("string")
                n3979 = call <vilib>:"System Exec.vi"("run minimized? (F)"=TRUE, "wait until completion? (T)"=TRUE, "working directory"=path "C:/LAB-IQ-NXT", "command line"="C:\\LAB-IQ-NXT\\JPostH.bat") -> ("standard error"=→"Respose From Server 2":string, "standard output"=w4961:string)  [unwired: 4 in, 2 out]
                "standard output 2" <- w4961
                n3980 = Match Pattern(string=w4961, regular expression="JSONH Check String") -> (match substring=w4959:string, offset past match=w4958:i32)  [unwired: 1 in, 2 out]
                n3981 = Equal?(x=w4959, y="JSONH Check String") -> (x = y?=→"Upload \nConfirmed 2":bool)
              }
            }
            n3982 = Divide(x=w4801, y=3600.0 ("f")) -> (x/y=w4794:dbl)
            n3983 = local read "run time"() -> (w4851:string[])
            n3984 = Round To Nearest(number=w4794) -> (nearest integer value=w4793:dbl)
            n3985 = Number To Decimal String(number=w4793) -> (decimal integer string=w4792:string)  [unwired: 1 in]
            n3986 = Index Array(array="Sensor Information", index (col) #1=0 ("disabled index (col)"), index (col) #2=1 ("index (col)"), index (col) #3=2 ("index (col)"), index (col) #4=3 ("index (col)")) -> (element #1=→"Sensor name":string[], element #2=→"model num":string[], element #3=→"run time":string[], element #4=→"state":string[])  [unwired: 4 in]
            n3987 = Insert Into Array(array=w4851, index=1, new element #1=w4792, new element #2=w4792, new element #3=w4792, new element #4=w4792, new element #5=w4792, new element #6=w4792) -> (w4816:string[])
            "run" <- w4816
            n3988 = local read "out"() -> (w4798:string[])
            n3989 = local read "Sensor Information"() -> (w4818:string[][])
            n3990 = Replace Array Subset(array=w4818, new element #1=w4816, index (col) #1=2 ("disabled index (col)"), new element #2=w4798, index (col) #2=3 ("index (col)")) -> (w4817:string[][])  [unwired: 2 in]
            n3991 = local write "Sensor Information"(w4817) -> ()
          }
        }
        n3992 = case shown="True" w4765 {
          frame False {
          }
          frame True {
            n3993 = Equal?(x="FLAG", y=0.0) -> (x = y?=w4782:bool)
            n3994 = case shown="False" w4782 {
              frame False {
                n3995 = Get Date/Time In Seconds() -> (seconds since 1Jan1904=w4788:timestamp)
                n3996 = local read "START 2"() -> (w4786:dbl)
                n3997 = To Double Precision Float(number=w4788) -> (double precision float=w4787:dbl)
                n3998 = Subtract(x=w4787, y=w4786) -> (x-y=→"SENSOR TIME  2":dbl)
              }
              frame True {
                n3999 = Get Date/Time In Seconds() -> (seconds since 1Jan1904=w4790:timestamp)
                n4000 = To Double Precision Float(number=w4790) -> (double precision float=→"START 2":dbl)
                n4001 = local write "FLAG"(100.0 ("FLAG")) -> ()
